vi "Vision Global Var..vi"() -> ()   [LabVIEW 2017]
panel:
  out "Kicker Y":dbl
  out "Kicker X":dbl
  out "Theta":dbl
  out "Energy":dbl
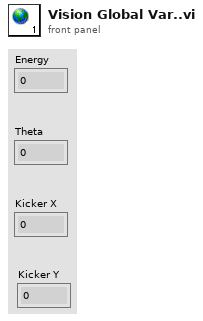
[diagram p1: front panel]
diagram:
